vi "uStringManipulation_DO.vi"(8 "error in (no error)":errorcluster, 10 "String in":string, 11 "uStringManipulation in":refnum<class "uStringManipulation.lvclass">) -> (0 "error out":errorcluster, 2 "String":string, 3 "uStringManipulation out":refnum<class "uStringManipulation.lvclass">)   [LabVIEW 2021, in "uFramework.lvlib" / "uStringManipulation.lvclass"]
doc: "This is the main method for manipulating the string. The default parent's behavior is to pass the string as-is. On error, it returns a blank string."
uses:
  uStringManipulation.lvclass
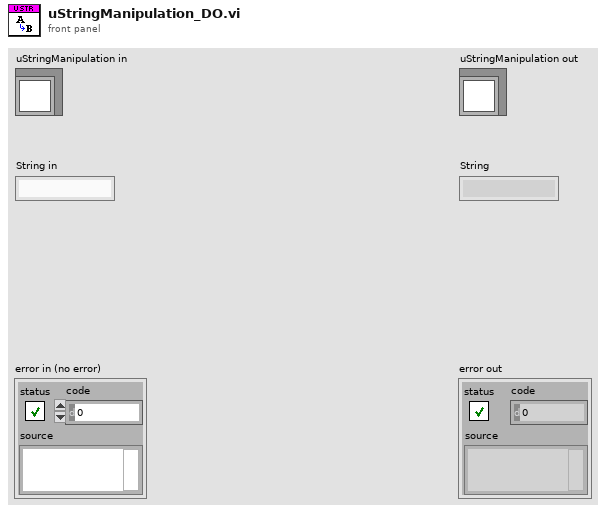
[diagram p1: front panel]
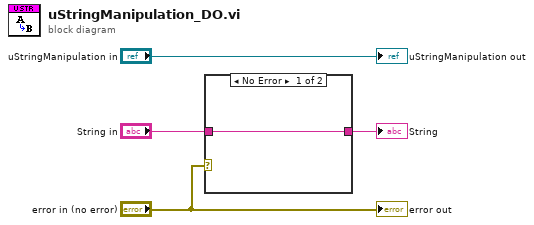
[diagram p0: block diagram]
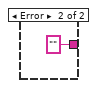
[diagram p2: hidden frame]
diagram:
  n1 = case shown="No Error" "error in (no error)" {
    tunnel: "String in" -> [w5 _]
    tunnel: [w5 "" ("String in")] -> w1
    frame No Error {
    }
    frame Error {
    }
  }
  "String" <- w1
  "error out" <- "error in (no error)"
  "uStringManipulation out" <- "uStringManipulation in"
